vi "niFPGA FFT Outside SCTL Permute Inputs.vi"(0 "input index":u16, 5 "K - 1":u8, 7 "K - 16":i8) -> (4 "mem block A?":bool, 6 "output address":u16, 8 "input address":u16)   [LabVIEW 2017]
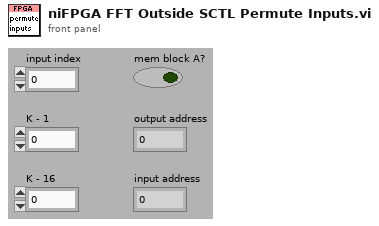
[diagram p1: front panel]
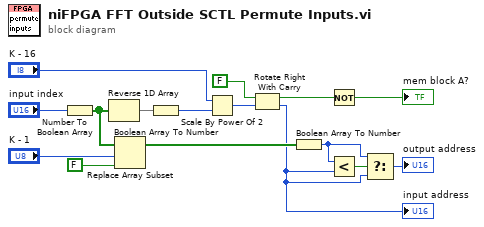
[diagram p0: block diagram]
diagram:
  n1 = Number To Boolean Array(number="input index") -> (Boolean array=w14:bool[])
  n2 = Reverse 1D Array(array=w14) -> (reversed array=w5:bool[])
  n3 = Replace Array Subset(array=w14, new element=FALSE ("new element/subarray"), index="K - 1") -> (w16:bool[])
  n4 = Boolean Array To Number(Boolean array=w5) -> (number=w6:u16)
  n5 = Scale By Power Of 2(n="K - 16", x=w6) -> (x*2^n=w9:u16)
  n6 = Rotate Right With Carry(2:w9, 3:FALSE ("carry")) -> (0:w11:u16, 1:w12:bool)
  "input address" <- w11
  n7 = Boolean Array To Number(Boolean array=w16) -> (number=w13:u16)
  n8 = Not(x=w12) -> (.not. x?=→"mem block A?":bool)
  n9 = Less?(x=w13, y=w11) -> (x < y?=w7:bool)
  n10 = Select(t=w13, s=w7, f=w11) -> (s? t:f=→"output address":u16)
